vi "Backup database.vi"(8 "error in (no error)":errorcluster, 10 "Destination":path, 11 "Source":path) -> (0 "error out":errorcluster)   [LabVIEW 2020, in "sqlite3.lvlib"]
uses:
  sqlite3.lvlib
  sqlite/subvi/Error Converter (ErrCode or Status).vi
  sqlite/VIs/errstr.vi
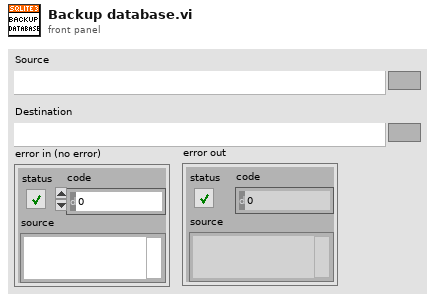
[diagram p1: front panel]
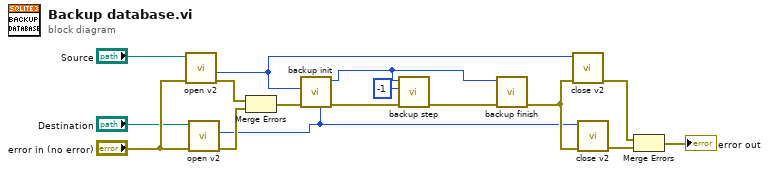
[diagram p0: block diagram]
diagram:
  n1 = call "open v2.vi"("error in (no error)"="error in (no error)", "filename"="Source") -> ("error out"=w12:errorcluster, "ppDb out"=w8:u64)  [unwired: 8 in]
  n2 = call "open v2.vi"("error in (no error)"="error in (no error)", "filename"="Destination") -> ("error out"=w11:errorcluster, "ppDb out"=w7:u64)  [unwired: 8 in]
  n3 = Merge Errors(w12, w11) -> (w10:errorcluster)
  n4 = call "backup init.vi"("ref dest"=w7, "error in (no error)"=w10, "ref src"=w8) -> ("error out"=w16:errorcluster, "backup_ref"=w14:u64)  [unwired: 7 in]
  n5 = call "backup step.vi"("error in (no error)"=w16, "page"=-1, "backup_ref"=w14) -> ("error out"=w15:errorcluster)  [unwired: 8 in]
  n6 = call "backup finish.vi"("error in (no error)"=w15, "backup_ref"=w14) -> ("error out"=w9:errorcluster)  [unwired: 9 in]
  n7 = call "close v2.vi"("error in (no error)"=w9, "para0"=w8) -> ("error out"=w4:errorcluster)  [unwired: 9 in]
  n8 = call "close v2.vi"("error in (no error)"=w9, "para0"=w7) -> ("error out"=w5:errorcluster)  [unwired: 9 in]
  n9 = Merge Errors(w4, w5) -> (→"error out":errorcluster)
